vi "Temp trig.vi"(8 "distance":dbl, 9 "angle (radian)":dbl, 10 "sensor x":dbl, 11 "sensor y":dbl) -> (2 "detected y":dbl, 3 "detected x":dbl)   [LabVIEW 2012]
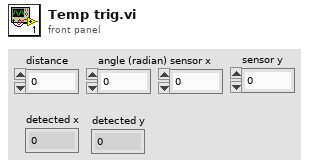
[diagram p1: front panel]
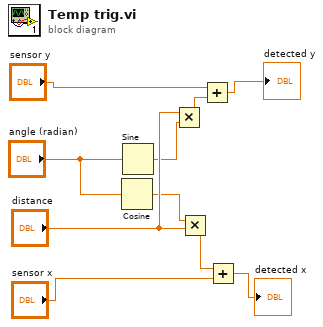
[diagram p0: block diagram]
diagram:
  n1 = Cosine(x="angle (radian)") -> (cos(x)=w2:dbl)
  n2 = Sine(x="angle (radian)") -> (sin(x)=w3:dbl)
  n3 = Multiply(x="distance", y=w3) -> (x*y=w8:dbl)
  n4 = Multiply(x=w2, y="distance") -> (x*y=w5:dbl)
  n5 = Add(x="sensor y", y=w8) -> (x+y=→"detected y":dbl)
  n6 = Add(x=w5, y="sensor x") -> (x+y=→"detected x":dbl)
